vi "Calibr WriteParam.vi"(8 "error in (no error)":errorcluster, 9 "intercept":dbl, 10 "slope":dbl) -> (0 "error out":errorcluster)   [LabVIEW 2018, in "Calibr.lvclass"]
uses:
  Calibr.lvclass
  Calibr.lvclass/Calibr.ctl
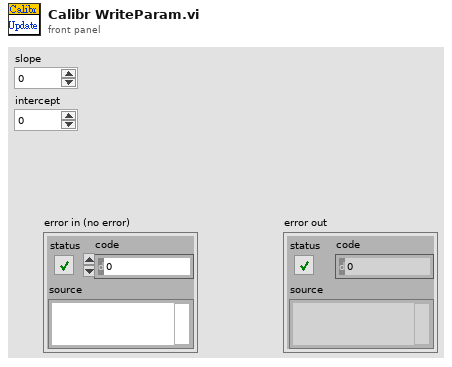
[diagram p1: front panel]
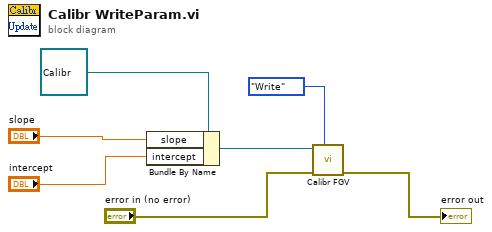
[diagram p0: block diagram]
diagram:
  n1 = Bundle By Name(cluster=refnum<class "Calibr.lvclass"> refnum ("Calibr in"), "slope"="slope", "intercept"="intercept") -> (w5:refnum<class "Calibr.lvclass">)
  n2 = call "Calibr FGV.vi"("Function"=enum16{"Init", "Read", "Write"}."Write", "error in (no error)"="error in (no error)", "Calibr in"=w5) -> ("error out"=→"error out":errorcluster)  [unwired: 7 in, 1 out]
